vi "In Aux Port.vi"(8 "error in (no error)":errorcluster, 10 "state":i32, 11 "port":i32) -> (0 "error out":errorcluster, 2 "state out":i32, 3 "function return":u32)   [LabVIEW 2014, in "atmcd32d.lvlib"]
doc: "unsigned int WINAPI InAuxPort(int port, int * state);"
uses:
  atmcd32d.lvlib
  atmcd32d.dll
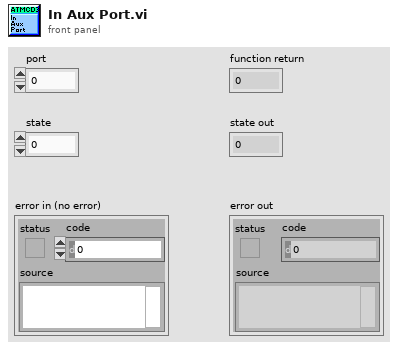
[diagram p1: front panel]
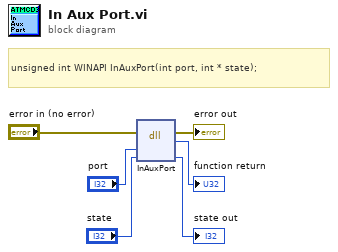
[diagram p0: block diagram]
diagram:
  # "unsigned int WINAPI InAuxPort(int port, int * state);"
  n1 = dll-call lib="C:/Users/Bakir/Documents/Lambda2-Testing/lib/Andorlib/atmcd32d.*" fn="InAuxPort"(error in="error in (no error)", "port"="port", "state"="state") -> (error out=→"error out":errorcluster, →"function return":u32, "state"=→"state out":i32)  [unwired: 3 in, 1 out]
